vi "Error Handler - Confirm Quit.vi"() -> (2 "exit confirmed":bool=TRUE)   [LabVIEW 2019]
doc: "Queries the user to find out if the application should exit or not."
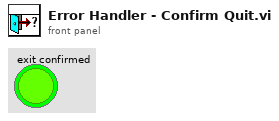
[diagram p1: front panel]
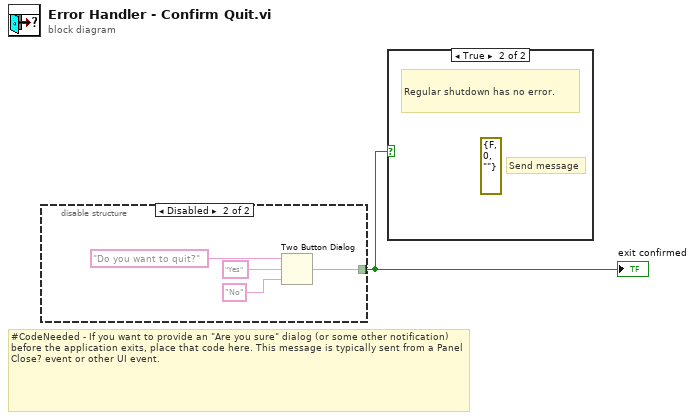
[diagram p0: block diagram]
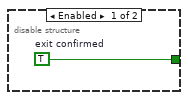
[diagram p3: hidden frame]
diagram:
  # "#CodeNeeded - If you want to provide an \"Are you sure\" dialog (or some other notification) before the application exits, place that code here. This message is typically sent from a Panel Close? event or other UI event."
  n1 = disable-structure shown="Disabled" {
    disable-tunnel: [w2 w3] -> w1
    frame Enabled {
      w2 = TRUE  # exit confirmed
    }
    frame Disabled {
      n2 = Two Button Dialog(message="Do you want to quit?" ("Do you want to quit?"), 1:"No" ("No"), 2:"Yes" ("Yes")) -> (T button?=w3:bool)
    }
  }
  "exit confirmed" <- w1
  n3 = case shown="True" w1 {
    frame False {
    }
    frame True {
      (unwired) errorcluster {"status"=FALSE, "code"=0, "source"=""} ("error IO")
      # "Send message"
      # "Regular shutdown has no error."
    }
  }
